vi "Data Sort.vi"(11 "Data Points (12 x65)(11x64)":dbl[][](array[numeric])) -> (2 "Data Points":T1(array[cluster]))   [LabVIEW 2017]
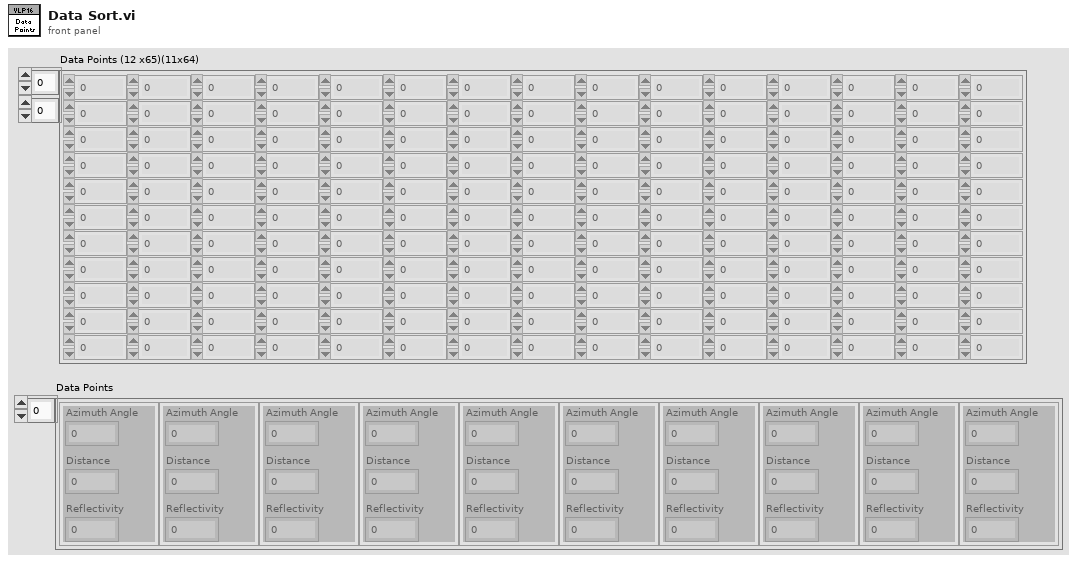
[diagram p1: front panel]
types:
  T1 = cluster{"Azimuth Angle":dbl, "Distance":dbl, "Reflectivity":dbl}[]
  T2 = cluster{"Numeric":dbl, "Numeric":dbl, "Numeric":dbl}
  T3 = cluster{"Numeric":dbl, "Numeric":dbl, "Numeric":dbl}[]
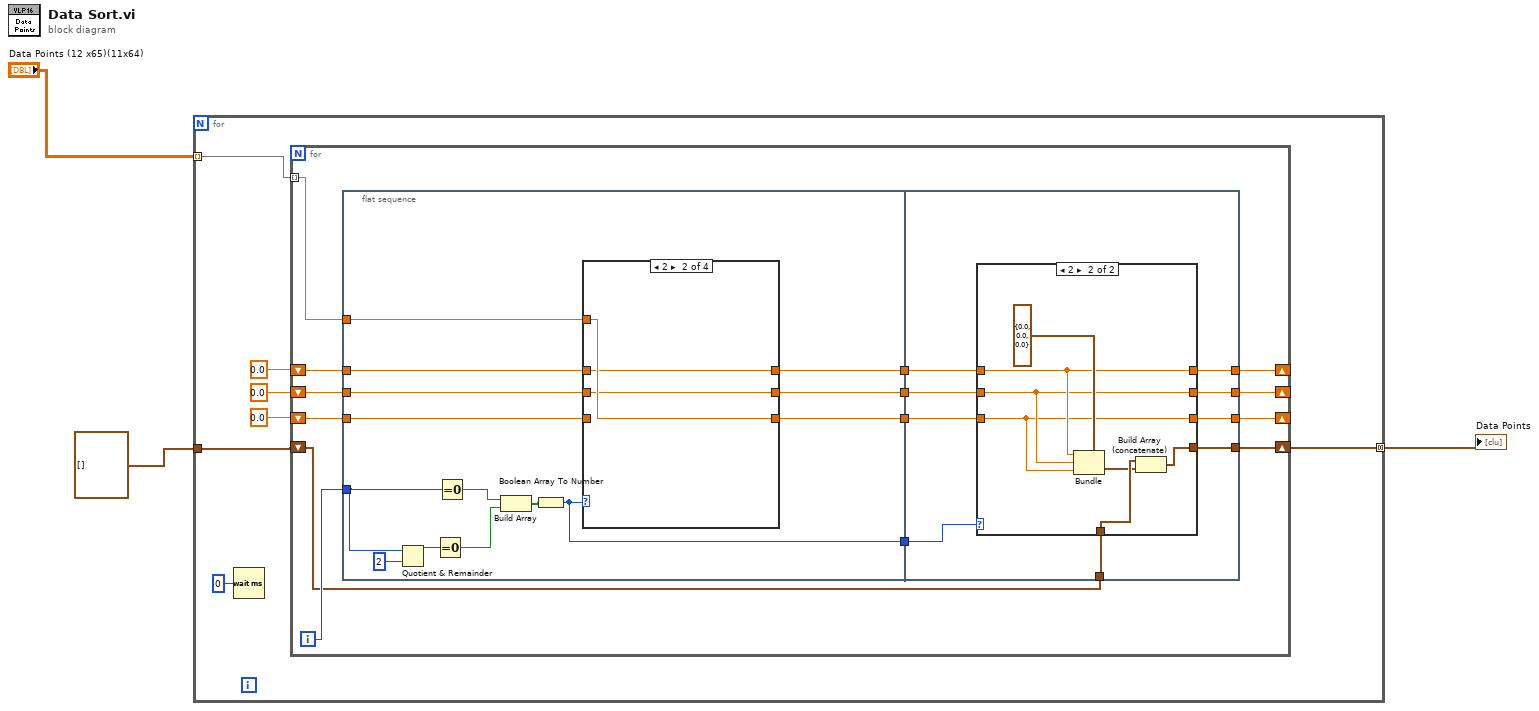
[diagram p0: block diagram]
diagram:
  n1 = for {
    tunnel: "Data Points (12 x65)(11x64)" -> [w10] mode=indexing
    tunnel: cluster{dbl, dbl, dbl}[] [] -> [w9]
    tunnel: [w4] -> w1 mode=concatenating
    n2 = Wait (ms)(milliseconds to wait=u32 0) -> ()  [unwired: 1 out]
    n3 = for {
      tunnel: w10 -> [w24] mode=indexing
      shift-right: [w11] -> w4
      shift-left: w9 -> [w12]
      shift-right: [w16] -> _
      shift-left: 0.0 -> [w23]
      shift-right: [w15] -> _
      shift-left: 0.0 -> [w22]
      shift-right: [w14] -> _
      shift-left: 0.0 -> [w21]
      i -> [w13]
      n4 = flat-sequence {
        tunnel: w13 -> [w38]
        tunnel: w24 -> [w32]
        tunnel: w23 -> [w31]
        tunnel: w22 -> [w30]
        tunnel: w21 -> [w29]
        tunnel: [w28] -> w20
        tunnel: [w27] -> w19
        tunnel: [w26] -> w18
        tunnel: [w25] -> w17
        tunnel: w20 -> [w58]
        tunnel: w19 -> [w56]
        tunnel: w18 -> [w54]
        tunnel: w17 -> [w59]
        tunnel: [w57] -> w16
        tunnel: [w55] -> w15
        tunnel: [w53] -> w14
        tunnel: w12 -> [w52]
        tunnel: [w51] -> w11
        frame #0 {
          n5 = Quotient & Remainder(x=w38, y=2) -> (x-y*floor(x/y)=w36:i32)  [unwired: 1 out]
          n6 = Equal To 0?(x=w36) -> (x = 0?=w34:bool)
          n7 = Equal To 0?(x=w38) -> (x = 0?=w35:bool)
          n8 = Build Array(w35, w34) -> (w33:bool[])
          n9 = Boolean Array To Number(Boolean array=w33) -> (number=w25:u32)
          n10 = case shown="2" w25 {
            tunnel: w32 -> [w41 w44 _ w50]
            tunnel: w31 -> [w40 w43 w47 _]
            tunnel: [w40 w43 w47 w50] -> w28
            tunnel: w30 -> [_ w42 w46 w49]
            tunnel: [w41 w42 w46 w49] -> w27
            tunnel: w29 -> [w39 _ w45 w48]
            tunnel: [w39 w44 w45 w48] -> w26
            frame 0 {
              # "Odd Number - Distance"
            }
            frame 2 {
            }
            frame Default {
            }
            frame 3 {
            }
          }
        }
        frame #1 {
          n11 = case shown="2" w59 {
            tunnel: w58 -> [w63 w66]
            tunnel: [w63 w66] -> w57
            tunnel: w56 -> [w62 w65]
            tunnel: [w62 w65] -> w55
            tunnel: w54 -> [w61 w64]
            tunnel: [w61 w64] -> w53
            tunnel: w52 -> [w60 w69]
            tunnel: [w60 w67] -> w51
            frame 0, Default {
            }
            frame 2 {
              n12 = Bundle(cluster=T2 {"Numeric"=0.0, "Numeric"=0.0, "Numeric"=0.0}, "Numeric"=w66, "Numeric"=w65, "Numeric"=w64) -> (w68:T2)
              n13 = Build Array (concatenate)(w69, w68) -> (w67:T3)
            }
          }
        }
      }
    }
  }
  "Data Points" <- w1
